vi "Set DH Convention.vi"(8 "error in (no error)":errorcluster, 10 "DH Convention":T1, 11 "serial arm in":refnum<class "NI_Robotics_Serial Robot Arm.lvclass">) -> (0 "error out":errorcluster, 3 "serial arm out":refnum<class "NI_Robotics_Serial Robot Arm.lvclass">)   [LabVIEW 2017, in "NI_Robotics_Serial Robot Arm.lvclass"]
uses:
  <vilib>/robotics/Kinematics/Robot/NI_Robotics_Serial Robot Arm.lvclass
  <vilib>/robotics/Kinematics/DH Convention.ctl
  <vilib>/robotics/Kinematics/Robot/NI_Robotics_Serial Robot Arm.lvclass/NI_Robotics_Serial Robot Arm.ctl
  <vilib>/robotics/Kinematics/NI_Kinematics.lvlib
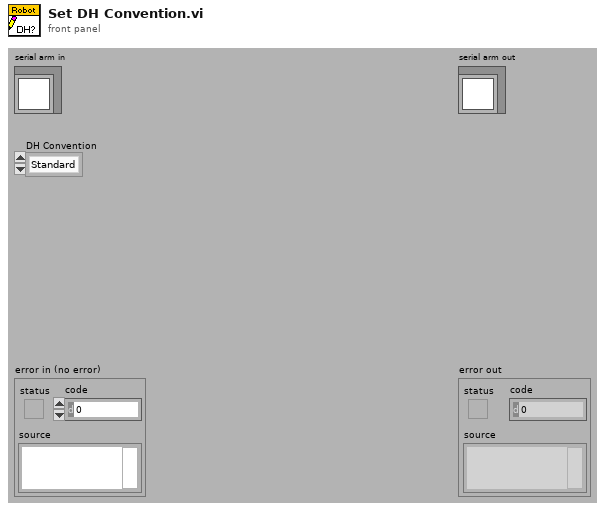
[diagram p1: front panel]
types:
  T1 = typedef "NI_Kinematics.lvlib/DH Convention.ctl" = enum16{"Standard", "Modified"}
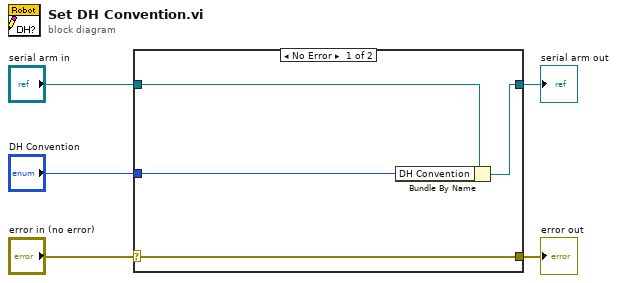
[diagram p0: block diagram]
diagram:
  n1 = case shown="No Error" "error in (no error)" {
    selector: "error in (no error)" -> [w9 w10]
    tunnel: [w9 w10] -> w4
    tunnel: [w7 w11] -> w2
    tunnel: "serial arm in" -> [w8 w11]
    tunnel: "DH Convention" -> [w6 _]
    frame No Error {
      n2 = Bundle By Name(cluster=w8, "DH Convention"=w6) -> (w7:refnum<class "NI_Robotics_Serial Robot Arm.lvclass">)
    }
    frame Error {
    }
  }
  "error out" <- w4
  "serial arm out" <- w2
